vi "LIA_FPGA-1a.vi"(1 "K":fxp<+,16,0>=0.001007080078125, 2 "nominal freq":fxp<+,16,0>=0.010009765625) -> (3 "phase (pi)":fxp<+/-,16,2>, 8 "ref":i16 format="%.0x", 9 "sig":i16 format="%.0x")   [LabVIEW 2012]
uses:
  <vilib>/rvi/DataTransferAndStorage/Container/Common/niFpgaContainerMetaDataKey.ctl
  <vilib>/rvi/DataTransferAndStorage/Container/Common/niFpgaContainerState.ctl
  <vilib>/rvi/DataTransferAndStorage/Container/Common/niFpgaDataTypeControl.ctl
  <vilib>/rvi/DataTransferAndStorage/Container/Common/niFpgaContainerImplementationControl.ctl
  <vilib>/rvi/DataTransferAndStorage/Container/Common/niFpgaContainerArbitrationOptionsControl.ctl
  <vilib>/rvi/DataTransferAndStorage/Container/Common/niFpgaTransferTypeControl.ctl
  <vilib>/rvi/DataTransferAndStorage/Container/Common/niFpgaContainerInitializationParameters.ctl
  <vilib>/rvi/Memory/Memory_Types/niFpgaMemoryInterfaceConfiguration.ctl
  <vilib>/rvi/FIFO/Fifo_Types/niFpgaFifoControlLogicControl.ctl
  <vilib>/Platform/TimedLoop/XDataNode/timing_clust.ctl
  <vilib>/Platform/TimedLoop/XDataNode/nitl_modes.ctl
  <vilib>/Platform/TimedLoop/XDataNode/wakeup.ctl
  <vilib>/rvi/FXPMathLib/FxpRectToPolar/subVIs/nifxpmath_RectToPolar_SimConfig.ctl
  <vilib>/rvi/DataTransferAndStorage/Container/Common/niFpgaContainerGetUniqueNameForEmu.vi
  <vilib>/rvi/DataTransferAndStorage/Container/Common/niFpgaContainerSetEmuInfo.vi
  <vilib>/rvi/eio/common/nirviEmuReportErrorAndStop.vi
  <vilib>/rvi/FXPMathLib/FxpRectToPolar/simVIs/DllFxpRectToPolarTemp_sub.vi
  <vilib>/rvi/Emulation/niFpgaSctlEmulationRegisterWithScheduler.vi
  <vilib>/rvi/FIFO/Fifo_Resource/nirvififoEmulationSetSize.vi
  <vilib>/rvi/Emulation/niFpgaSctlEmulationFifoFullMgr.vi
  <vilib>/rvi/errors/niFpgaSetErrorForExecOnDevCompSimple.vi
  <vilib>/rvi/Emulation/niFpgaSctlEmulationScheduler.vi
  <vilib>/rvi/eio/common/nirviEmuTemplateMethod_errors.vi
  <vilib>/rvi/Emulation/niFpgaSctlEmulationGetInTimedLoop.vi
  <vilib>/rvi/Emulation/niFpgaSctlEmulationResourceMgr.vi
  <vilib>/rvi/LocalResourceManager/LocalResourceManager.xnode
  <vilib>/Platform/TimedLoop/XDataNode/XDataNode.xnode
  <vilib>/rvi/FXPMathLib/FxpRectToPolar/XNode/nifxpmath_RectToPolar.xnode
  <vilib>/rvi/DataTransferAndStorage/Container/XNode/niFpgaContainer.xnode
  <vilib>/rvi/FIFO/Fifo_Resource/nirvififoEmulationRead.vi
  <vilib>/rvi/FXPMathLib/FxpInterpret/XNode/nifxpmath_Interpret.xnode
  <vilib>/eio/EIONode/EIONode.xnode
  <vilib>/rvi/FIFO/Fifo_Resource/nirvififoEmulationWrite.vi
  <vilib>/Platform/TimedLoop/XDataNode/XDNodeRunTimeDep.lvlib
panel:
  out "Nominal Freq":fxp<+/-,64,32>
  in  "stop 2":bool
  in  "Filter Constant":i64
  in  "Period":u16=1000
  out "ticks":u16
  out "channelQ":i64
  out "channelI":i64
  out "f":fxp<+/-,32,0> format="%.32g"
  in  "start":bool
  in  "dec2":i16=1
  in  "dec1":i16=1
  in  "stages":i8=1
  in  "stop":bool
  in  "decimation":i16=1024
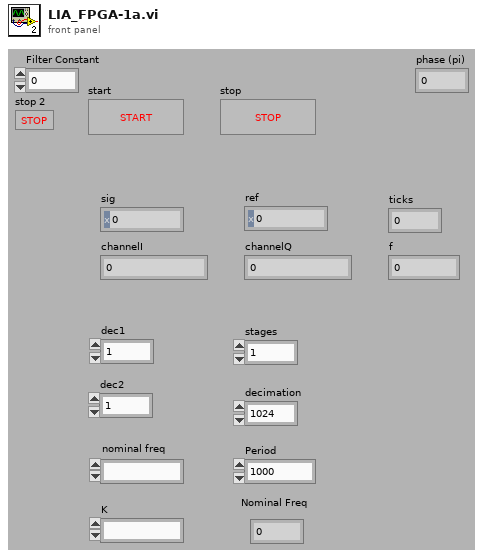
[diagram p1: front panel]
types:
  T1 = typedef "XDNodeRunTimeDep.lvlib/timing_clust.ctl" = cluster{"Expected End [f-1]":u64, "Actual End [f-1]":u64, "Finished Late? [f-1]":bool, "Expected End [i-1]":u64, "Actual End [i-1]":u64, "Finished Late? [i-1]":bool, "Expected Start [i]":u64, "Actual Start [i]":u64, "Expected Start [f]":u64, "Actual Start [f]":u64, "Source Name":string, "Structure Name":string, "Period":i64, "Deadline":i64, "Offset":i64, "Start":i64, "Priority":i32, "Timeout":i32, "Mode":T2, "Wakeup Reason":T3, "Error":errorcluster, "Source Type":string, "Secondary Source Type":string, "Global End Time":u64, "Global Start Time":u64, "Frame Duration":u64, "Iteration Duration":u64, "Assigned CPU":i32, "I/O Scan Engine Mode":u32}
  T2 = typedef "XDNodeRunTimeDep.lvlib/nitl_modes.ctl" = enum32{"No Change", "Process missed periods, maintain original phase", "Discard missed periods, maintain original phase", "Process missed periods, ignore original phase", "Discard missed periods, ignore original phase"}
  T3 = typedef "XDNodeRunTimeDep.lvlib/wakeup.ctl" = enum32{"Normal", "Aborted", "Asynchronous wakeup", "Timing source error", "Timed loop error", "Timeout"}
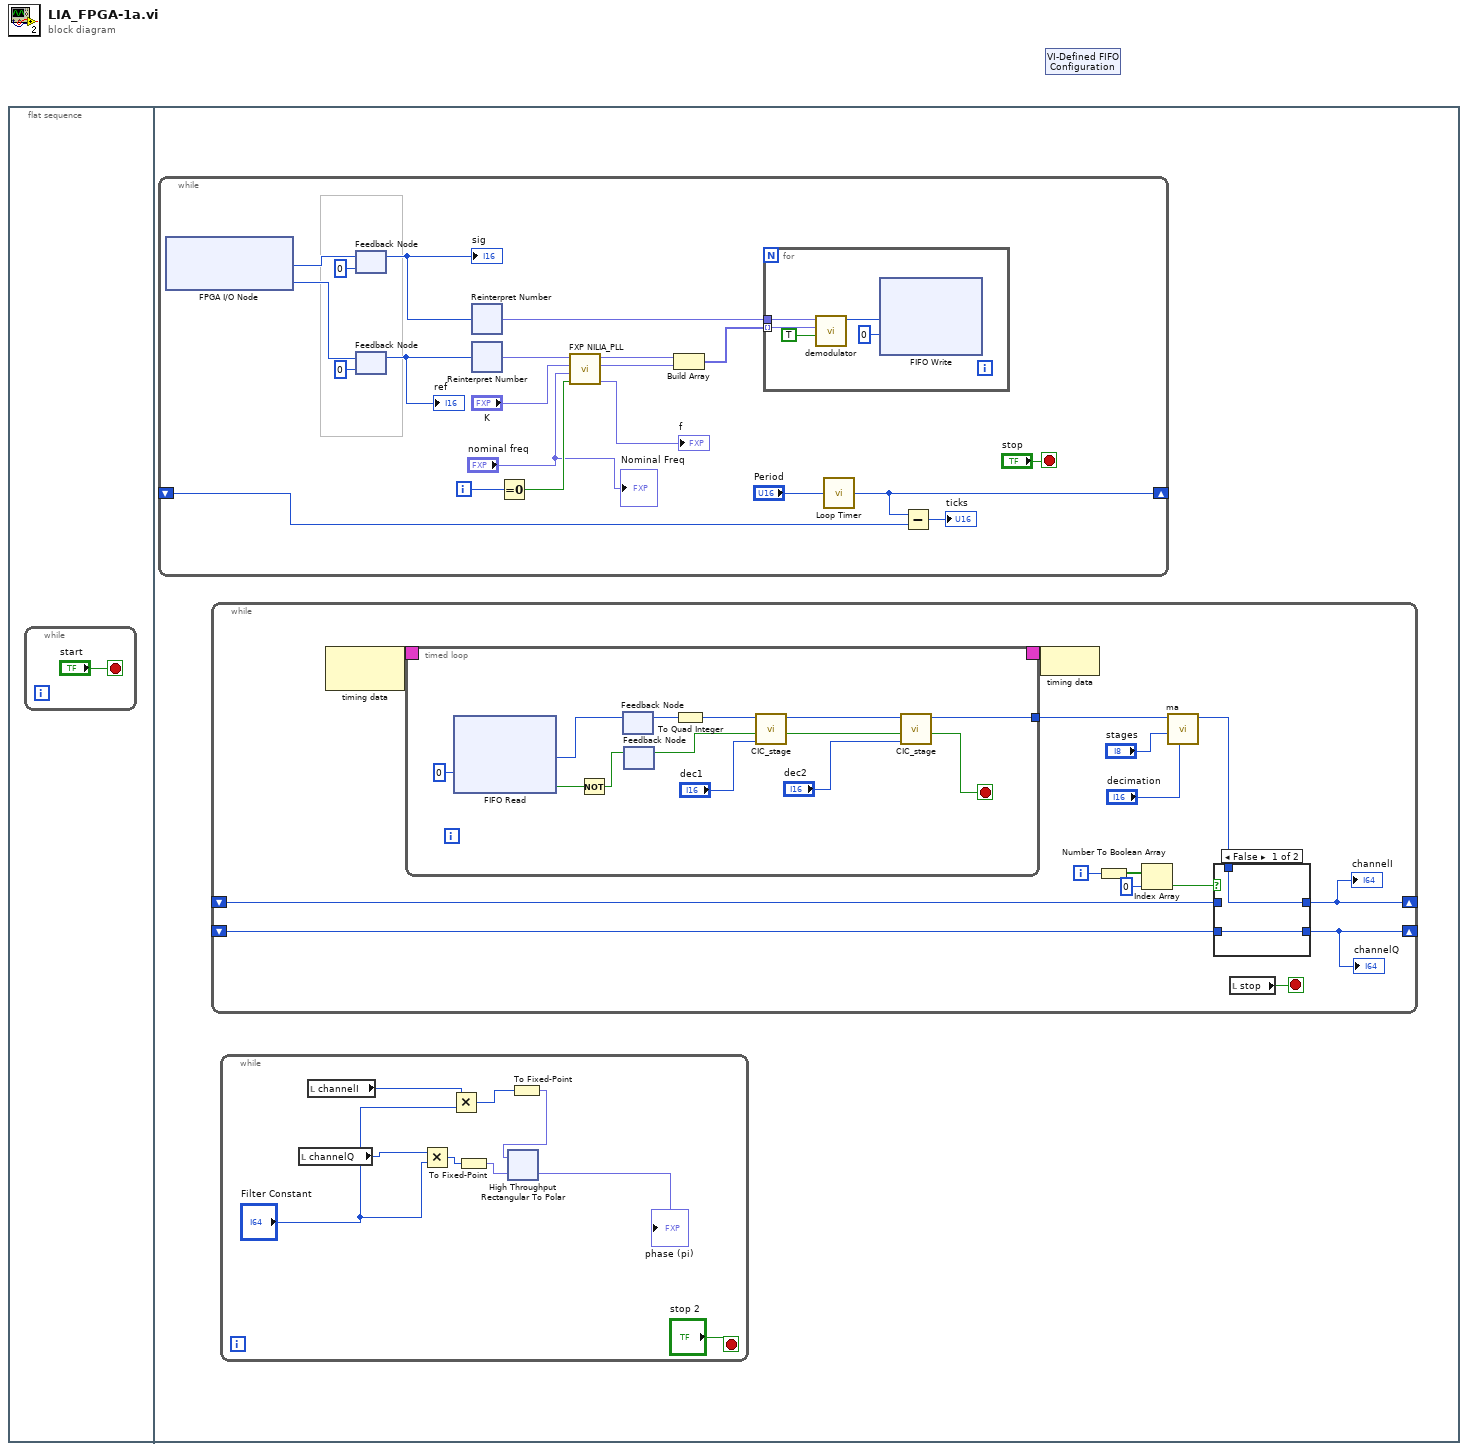
[diagram p0: block diagram]
diagram:
  n1 = flat-sequence {
    frame #0 {
      n2 = while {
        stop <- "start" stop-if-true
      }
    }
    frame #1 {
      n3 = while {
        shift-right: [w65] -> _
        shift-left: _ -> [w64]
        i -> [w68]
        stop <- "stop" stop-if-true
        n4 = xnode "FPGA I/O Node"() -> ("Connector0/AI6"=w58:i16, "Connector0/AI7"=w55:i16)  [unwired: 2 in, 2 out]
        n5 = feedback #1(i16 0 ("y")) -> (w57:i16)
        "sig" <- w57
        n6 = feedback-in #1(w58) -> ()
        n7 = feedback #2(i16 0 ("z [I32.1]")) -> (w56:i16)
        "ref" <- w56
        n8 = feedback-in #2(w55) -> ()
        n9 = xnode "Reinterpret Number"("x"=w57) -> ("y"=w61:fxp<+/-,16,1>)
        n10 = xnode "Reinterpret Number"("x"=w56) -> ("y"=w54:fxp<+/-,16,1>)
        n11 = Equal To 0?(x=w68) -> (x = 0?=w49:bool)
        n12 = call "FXP NILIA_PLL.vi"("reset?"=w49, "norminal freq [U16.0]"="nominal freq", "alpha [U16.0]"="K", "x[I16.1]"=w54) -> ("f"=→"f":fxp<+/-,32,0>, "sin(z)"=w51:fxp<+/-,16,2>, "cos(z)"=w50:fxp<+/-,16,2>)  [unwired: 4 in, 1 out]
        n13 = Build Array(w50, w51) -> (w62:fxp<+/-,16,2>[])
        n14 = for {
          tunnel: w61 -> [w71]
          tunnel: w62 -> [w69] mode=indexing
          n15 = call "demodulator.vi"("New Data"=TRUE, "ref"=w69, "signal"=w71) -> ("x*y"=w72:i32)  [unwired: 8 out]
          n16 = xnode ("FIFO Write")("Element"=w72, "Timeout"=0) -> ()  [unwired: 1 in, 2 out]
        }
        n17 = call "Loop Timer"("Count(Ticks)"="Period") -> ("Tick Count(Ticks)"=w65:u16)
        n18 = Subtract(x=w65, y=w64) -> (x-y=→"ticks":u16)
        "Nominal Freq" <- "nominal freq"
      }
      n19 = while {
        shift-right: [w75] -> _
        shift-left: _ -> [w77]
        shift-right: [w74] -> _
        shift-left: _ -> [w76]
        i -> [w82]
        stop <- w84 stop-if-true
        n20 = node-c288() -> (w88:T1)  [unwired: 1 out]
        n21 = timed-loop {
          timing: w88 -> [_]
          timing-out: [_] -> w87
          tunnel: [w96] -> w83
          stop <- w95 stop-if-true
          n22 = xnode ("FIFO Read")("Timeout"=0) -> ("Element"=w103:i32, "Timed Out?"=w102:bool)  [unwired: 1 in, 1 out]
          n23 = Not(x=w102) -> (.not. x?=w101:bool)
          n24 = feedback-in #3(w103) -> ()
          n25 = feedback #3() -> (w105:i32)  [unwired: 1 out]
          n26 = feedback-in #4(w101) -> ()
          n27 = feedback #4() -> (w99:bool)  [unwired: 1 out]
          n28 = To Quad Integer(1:w105) -> (0:w100:i64)
          n29 = call "CIC_stage.vi"("decimate factor"="dec1", "New Data"=w99, "input"=w100) -> ("Data Ready"=w97:bool, "output"=w98:i64)  [unwired: 7 out]
          n30 = call "CIC_stage.vi"("decimate factor"="dec2", "New Data"=w97, "input"=w98) -> ("Data Ready"=w95:bool, "output"=w96:i64)  [unwired: 7 out]
        }
        n31 = node-c288(w87) -> ()
        n32 = Number To Boolean Array(number=w82) -> (Boolean array=w81:bool[])
        n33 = Index Array "Index Array"(array=w81, index=0) -> (element=w79:bool)
        n34 = call "ma.vi"("decimate"="decimation", "stages"="stages", "input"=w83) -> ("output"=w78:i64)  [unwired: 8 out]
        n35 = case shown="False" w79 {
          tunnel: w78 -> [w90 w92]
          tunnel: [w90 w91] -> w75
          tunnel: [w89 w92] -> w74
          tunnel: w77 -> [_ w91]
          tunnel: w76 -> [w89 _]
          frame False {
          }
          frame True {
          }
        }
        "channelI" <- w75
        "channelQ" <- w74
        n36 = local read "stop"() -> (w84:bool)
      }
      n37 = while {
        stop <- "stop 2" stop-if-true
        n38 = local read "channelQ"() -> (w9:i64)
        n39 = local read "channelI"() -> (w10:i64)
        n40 = Multiply(x=w9, y="Filter Constant") -> (x*y=w5:i64)
        n41 = Multiply(x=w10, y="Filter Constant") -> (x*y=w7:i64)
        n42 = To Fixed-Point(number=w5) -> (fixed-point=w4:fxp<+/-,64,64>)  [unwired: 1 in]
        n43 = To Fixed-Point(number=w7) -> (fixed-point=w6:fxp<+/-,64,64>)  [unwired: 1 in]
        n44 = xnode "High Throughput Rectangular To Polar"("x"=w6, "y"=w4) -> ("phase (pi)"=→"phase (pi)":fxp<+/-,16,2>)  [unwired: 1 out]
      }
    }
  }
  n45 = xnode "VI-Defined FIFO Configuration"() -> ()  [unwired: 1 out]
